vi "Save_data.vi"(11 "Data":waveform(dbl)[](array[waveform])) -> ()   [LabVIEW 2023]
uses:
  <vilib>/Utility/file.llb/Write Delimited Spreadsheet (DBL).vi
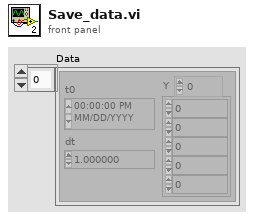
[diagram p1: front panel]
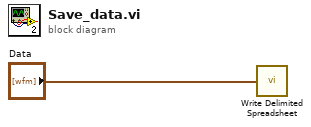
[diagram p0: block diagram]
diagram:
  n1 = call-poly <vilib>:"Write Delimited Spreadsheet.vi"("1D data"="Data") -> ()  [unwired: 13 in, 2 out]
